vi "Do.vi"(8 "error in (no error)":errorcluster, 10 "Actor in":refnum<class "Actor.lvclass">, 11 "Perform Action on Target Msg":refnum<class "Perform Action on Target Msg.lvclass">) -> (0 "error out":errorcluster, 2 "Actor out":refnum<class "Actor.lvclass">)   [LabVIEW 2024, in "ISeries Actor.lvlib" / "Perform Action on Target Msg.lvclass"]
doc: "This VI delivers the message to the actor by calling the appropriate method(s) on the actor."
uses:
  Perform Action on Target Msg.lvclass
  Perform Action on Target Msg.lvclass/Perform Action on Target Msg.ctl
  c33e8600-9278-4f06-b4d3-5d11a788da6f.vi
  ISeries Actor/ISeries Actor.lvclass
  <vilib>/ActorFramework/Actor/Actor.lvclass
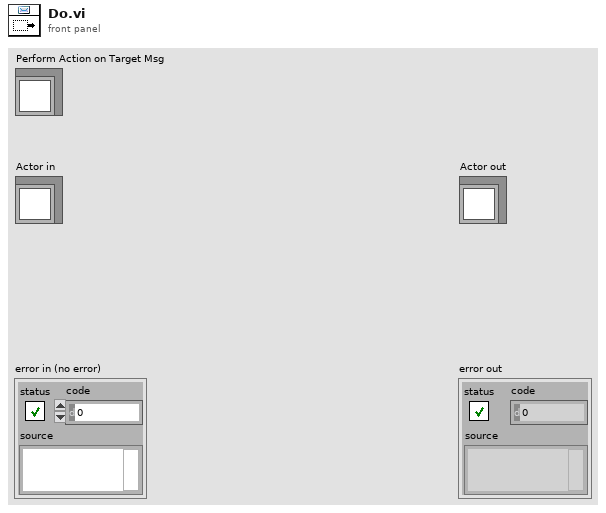
[diagram p1: front panel]
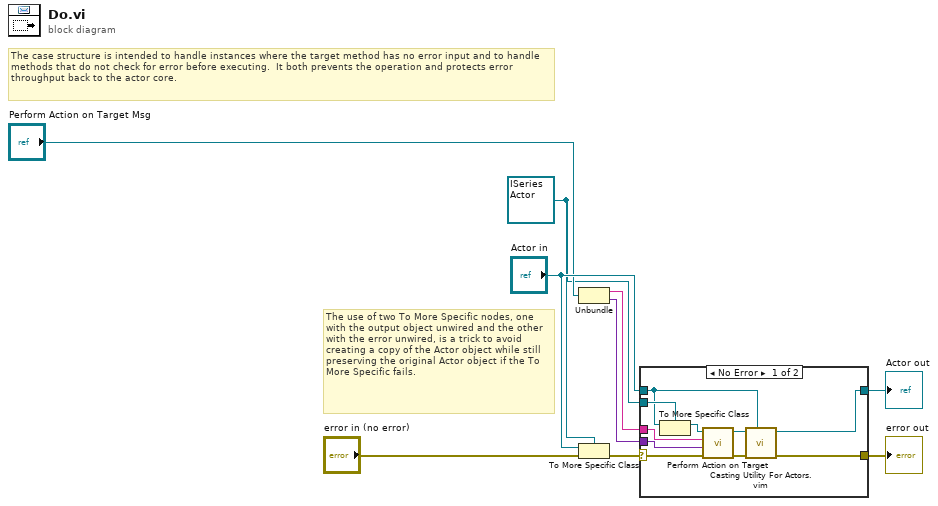
[diagram p0: block diagram]
diagram:
  w4 = refnum<class "ISeries Actor.lvclass"> refnum ("Actor in")
  # "The use of two To More Specific nodes, one with the output object unwired and the other with the error unwired, is a trick to avoid creating a copy of the Actor object while still preserving the original Actor object if the To More Specific fails."
  # "The case structure is intended to handle instances where the target method has no error input and to handle methods that do not check for error before executing.  It both prevents the operation and protects error throughput back to the actor core."
  n1 = Unbundle("Perform Action on Target Msg") -> (w2:string, w1:variant)
  n2 = To More Specific Class(target class=w4, reference="Actor in", error in="error in (no error)") -> (error out=w3:errorcluster)  [unwired: 1 out]
  n3 = case shown="No Error" w3 {
    selector: w3 -> [w19 w21]
    tunnel: [w13 w21] -> w9
    tunnel: [w14 w20] -> w8
    tunnel: "Actor in" -> [w16 w20]
    tunnel: w4 -> [w17 _]
    tunnel: w2 -> [w11 _]
    tunnel: w1 -> [w10 _]
    frame No Error {
      n4 = To More Specific Class(target class=w17, reference=w16) -> (specific class reference=w18:refnum<class "ISeries Actor.lvclass">)  [unwired: 1 in, 1 out]
      n5 = call-dynamic "Perform Action on Target.vi"("error in"=w19, "Input"=w10, "Task-Point Ident"=w11, "ISeries Actor in"=w18) -> ("error out"=w12:errorcluster, "ISeries Actor out"=w15:refnum<class "ISeries Actor.lvclass">)  [unwired: 6 in]
      n6 = call "Casting Utility For Actors.vim"("type"=w16, "error in (no error)"=w12, "Actor in"=w15) -> ("error out"=w13:errorcluster, "Actor out"=w14:refnum<class "Actor.lvclass">)  [unwired: 7 in]
    }
    frame Error {
      # "If type check fails, pass the original object out again."
    }
  }
  "error out" <- w9
  "Actor out" <- w8
